vi "detect modules.vi"(8 "error in":errorcluster, 10 "module in":refnum<class "Module.lvclass">, 11 "chassis in":refnum<class "Chassis.lvclass">) -> (0 "error out":errorcluster, 2 "module out":refnum<class "Module.lvclass">, 3 "chassis out":refnum<class "Chassis.lvclass">)   [LabVIEW 2014, in "SMI.lvlib" / "Module.lvclass"]
uses:
  Module.lvclass
  Chassis/Chassis.lvclass
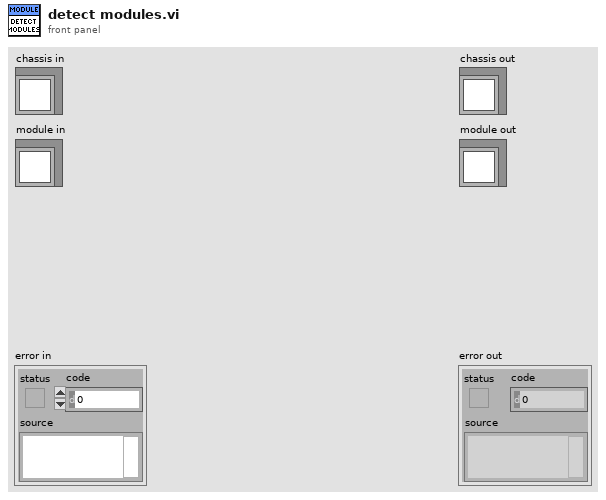
[diagram p1: front panel]
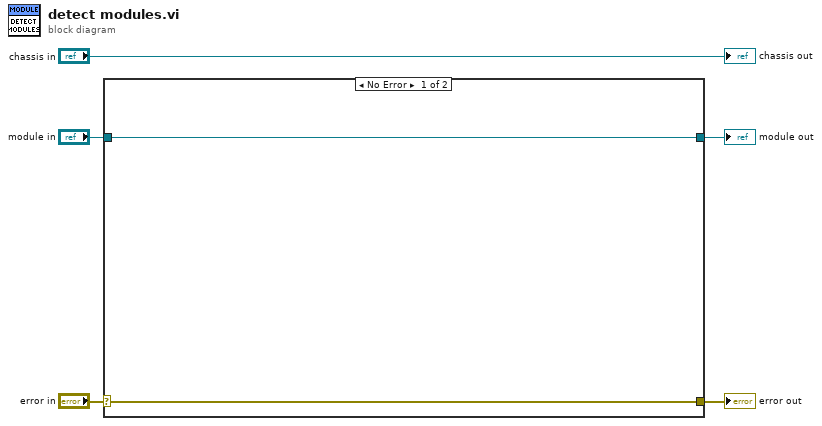
[diagram p0: block diagram]
diagram:
  n1 = case shown="No Error" "error in" {
    selector: "error in" -> [w6 w9]
    tunnel: [w6 w9] -> w4
    tunnel: [w7 w8] -> w2
    tunnel: "module in" -> [w7 w8]
    frame No Error {
    }
    frame Error {
    }
  }
  "error out" <- w4
  "module out" <- w2
  "chassis out" <- "chassis in"
